vi "DeviceOff.vi"(8 "error in (no error)":errorcluster, 11 "NHRDCModel in":refnum<class "NHRDCModel.lvclass">) -> (0 "error out":errorcluster, 3 "NHRDCModel out":refnum<class "NHRDCModel.lvclass">)   [LabVIEW 2018, in "AcPwrPlugins.lvlib" / "NHRDCModel.lvclass"]
doc: "This VI disables the instruments output form either generating or receiving a signal."
uses:
  NHRDCModel.lvclass
  AcPwrBaseClass/AcPwrBase.lvclass
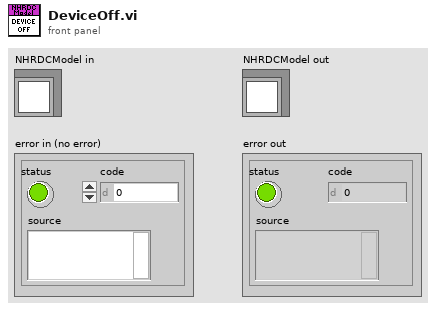
[diagram p1: front panel]
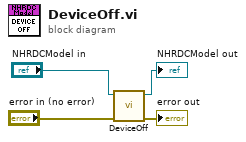
[diagram p0: block diagram]
diagram:
  n1 = call-parent "DeviceOff.vi"("error in (no error)"="error in (no error)", "AcPwrBase in"="NHRDCModel in") -> ("error out"=→"error out":errorcluster, "AcPwrBase out"=→"NHRDCModel out":refnum<class "NHRDCModel.lvclass">)  [unwired: 8 in]
